vi "Utility Read From Register - Float or Int.vi"(0 "VISA resource name":refnum<visa-resource-name>, 1 "Unit Address (1)":u8=1, 5 "Register Address (0)":u16, 9 "Num Of Reg (1)":u16=1 min=1 step=1, 11 "error in (no error)":errorcluster) -> (4 "VISA resource name out":refnum<visa-resource-name>, 6 "Data":sgl[](array[numeric]), 15 "error out":errorcluster)   [LabVIEW 2010, in "Eurotherm 32xx Series.lvlib"]
doc: "This VI reads value from specified registers of specified unit."
uses:
  <instrlib>/Eurotherm 32xx Series/Eurotherm 32xx Series.lvlib
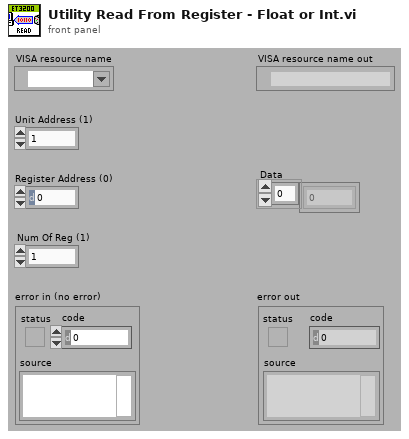
[diagram p1: front panel]
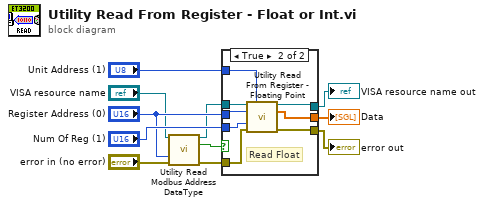
[diagram p0: block diagram]
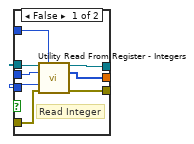
[diagram p2: hidden frame]
diagram:
  n1 = call <instrlib>:"Utility Read Modbus Address DataType.vi"("VISA resource name"="VISA resource name", "Register Address (0)"="Register Address (0)", "error in (no error)"="error in (no error)") -> ("VISA resource name out"=w2:refnum<visa-resource-name>, "Float32 (T)"=w7:bool, "error out"=w4:errorcluster)  [unwired: 9 in, 1 out]
  n2 = case shown="True" w7 {
    tunnel: w2 -> [w19 w25]
    tunnel: w4 -> [w18 w24]
    tunnel: [w17 w27] -> w11
    tunnel: "Unit Address (1)" -> [w16 w21]
    tunnel: "Register Address (0)" -> [w15 w22]
    tunnel: "Num Of Reg (1)" -> [w14 w23]
    tunnel: [w13 w26] -> w8
    tunnel: [w12 w20] -> w1
    frame False {
      # "Read Integer"
      n3 = call <instrlib>:"Utility Read From Register - Integers.vi"("VISA resource name"=w19, "Unit Address (1)"=w16, "Register Address (0)"=w15, "Num Of Reg (1)"=w14, "error in (no error)"=w18) -> ("VISA resource name out"=w17:refnum<visa-resource-name>, "Data"=w12:i16[], "error out"=w13:errorcluster)  [unwired: 8 in]
    }
    frame True {
      # "Read Float"
      n4 = call <instrlib>:"Utility Read From Register - Floating Point.vi"("VISA resource name"=w25, "Unit Address (1)"=w21, "Register Address (0)"=w22, "Num Of Reg (1)"=w23, "error in (no error)"=w24) -> ("VISA resource name out"=w27:refnum<visa-resource-name>, "Data"=w20:sgl[], "error out"=w26:errorcluster)  [unwired: 8 in]
    }
  }
  "VISA resource name out" <- w11
  "error out" <- w8
  "Data" <- w1
